vi "New Power Plant.vi"(11 "EV3 in":T1) -> (3 "EV3 out":T1)   [LabVIEW 2016]
uses:
  <vilib>/NXT/Subs/LVHSConnector.ctl
  <vilib>/NXT/LegoClasses/BrickReference/BrickReference.lvclass
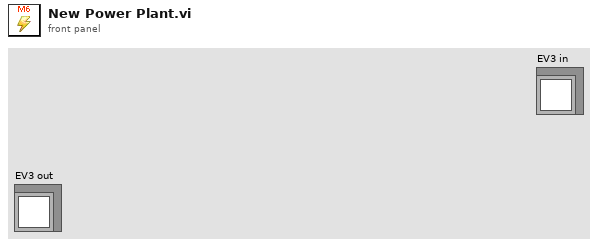
[diagram p1: front panel]
types:
  T1 = typedef "LVHSConnector.ctl" = refnum<class "BrickReference.lvclass">
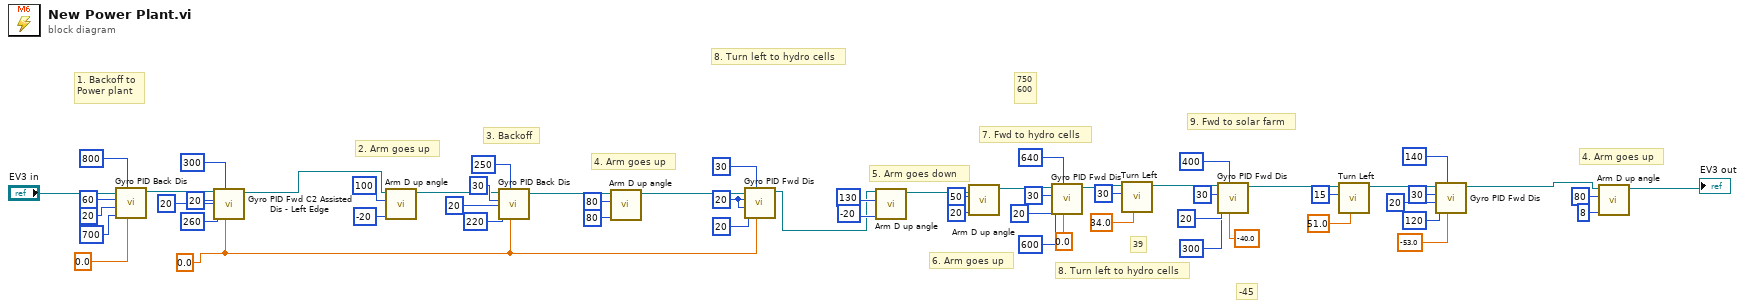
[diagram p0: block diagram]
diagram:
  w4 = 20 ("Max. speed")
  w3 = sgl 0.0 ("Target angle")
  # "8. Turn left to hydro cells"
  # "-45"
  # "39"
  # "750\n600"
  # "4. Arm goes up"
  # "9. Fwd to solar farm"
  # "8. Turn left to hydro cells"
  # "7. Fwd to hydro cells"
  # "6. Arm goes up"
  # "5. Arm goes down"
  # "4. Arm goes up"
  # "3. Backoff"
  # "2. Arm goes up"
  # "1. Backoff to\nPower plant"
  n1 = call "Gyro PID Back Dis.vi"("Target angle"=sgl 0.0, "Threshold to stop"=800, "Threshold to slow"=700, "Min. speed"=20, "Max. speed"=60, "EV3 in"="EV3 in") -> ("EV3 out"=w28:T1)  [unwired: 5 in]
  n2 = call "Gyro PID Fwd C2 Assisted Dis - Left Edge.vi"("Target angle"=w3, "Threshold to Stop"=300, "Threshold to slow"=260, "Min. speed"=20, "Max. speed"=20, "EV3 in"=w28) -> ("EV3 out"=w27:T1)  [unwired: 5 in]
  n3 = call "Arm D up angle.vi"("Power"=i8 -20, "Rotation"=100, "EV3 in"=w27) -> ("EV3 out"=w51:T1)  [unwired: 8 in]
  n4 = call "Gyro PID Back Dis.vi"("Target angle"=w3, "Threshold to stop"=250, "Threshold to slow"=220, "Min. speed"=20, "Max. speed"=30, "EV3 in"=w51) -> ("EV3 out"=w48:T1)  [unwired: 5 in]
  n5 = call "Arm D up angle.vi"("Power"=i8 80, "Rotation"=80, "EV3 in"=w48) -> ("EV3 out"=w6:T1)  [unwired: 8 in]
  n6 = call "Gyro PID Fwd Dis.vi"("Target angle"=w3, "Threshold to stop"=30, "Threshold to slow"=20, "Min. speed"=w4, "Max. speed"=w4, "EV3 in"=w6) -> ("EV3 out"=w5:T1)  [unwired: 5 in]
  n7 = call "Arm D up angle.vi"("Power"=i8 -20, "Rotation"=130, "EV3 in"=w5) -> ("EV3 out"=w44:T1)  [unwired: 8 in]
  n8 = call "Arm D up angle.vi"("Power"=i8 20, "Rotation"=50, "EV3 in"=w44) -> ("EV3 out"=w43:T1)  [unwired: 8 in]
  n9 = call "Gyro PID Fwd Dis.vi"("Target angle"=sgl 0.0, "Threshold to stop"=640, "Threshold to slow"=600, "Min. speed"=20, "Max. speed"=30, "EV3 in"=w43) -> ("EV3 out"=w37:T1)  [unwired: 5 in]
  n10 = call "Turn Left.vi"("Turning angle"=sgl 34.0, "Motor B (right)"=i8 30, "EV3 in"=w37) -> ("EV3 out"=w29:T1)  [unwired: 8 in]
  n11 = call "Gyro PID Fwd Dis.vi"("Target angle"=sgl -40.0, "Threshold to stop"=400, "Threshold to slow"=300, "Min. speed"=20, "Max. speed"=30, "EV3 in"=w29) -> ("EV3 out"=w21:T1)  [unwired: 5 in]
  n12 = call "Turn Left.vi"("Turning angle"=sgl 51.0, "Motor B (right)"=i8 15, "EV3 in"=w21) -> ("EV3 out"=w18:T1)  [unwired: 8 in]
  n13 = call "Gyro PID Fwd Dis.vi"("Target angle"=sgl -53.0, "Threshold to stop"=140, "Threshold to slow"=120, "Min. speed"=20, "Max. speed"=30, "EV3 in"=w18) -> ("EV3 out"=w15:T1)  [unwired: 5 in]
  n14 = call "Arm D up angle.vi"("Power"=i8 8, "Rotation"=80, "EV3 in"=w15) -> ("EV3 out"=→"EV3 out":T1)  [unwired: 8 in]
